vi "Target Startup Value Check.vi"(8 "error in (no error)":errorcluster) -> (0 "Ok to run?":bool)   [LabVIEW 2018]
panel:
  out "GRF Gain":bool
  out "Max Current":bool
  out "PCA weights":bool
  out "Logging Filename":bool
  out "Logging duration":bool
  out "Period Time":bool
  out "Bias":bool
  out "Current Rate":bool
  out "Mass":bool
  out "fc":bool
  out "HSD dF Thr":bool
  out "HSD F Thr":bool
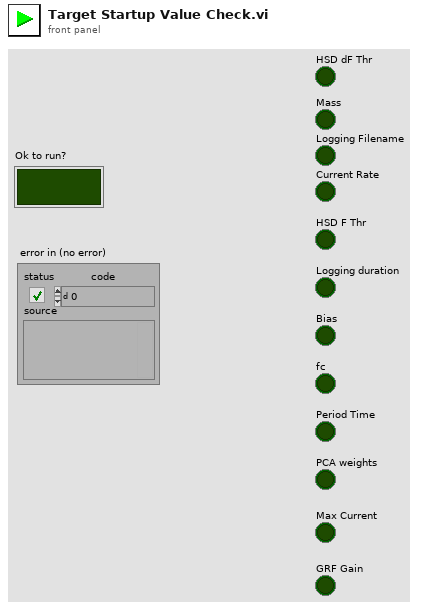
[diagram p1: front panel]
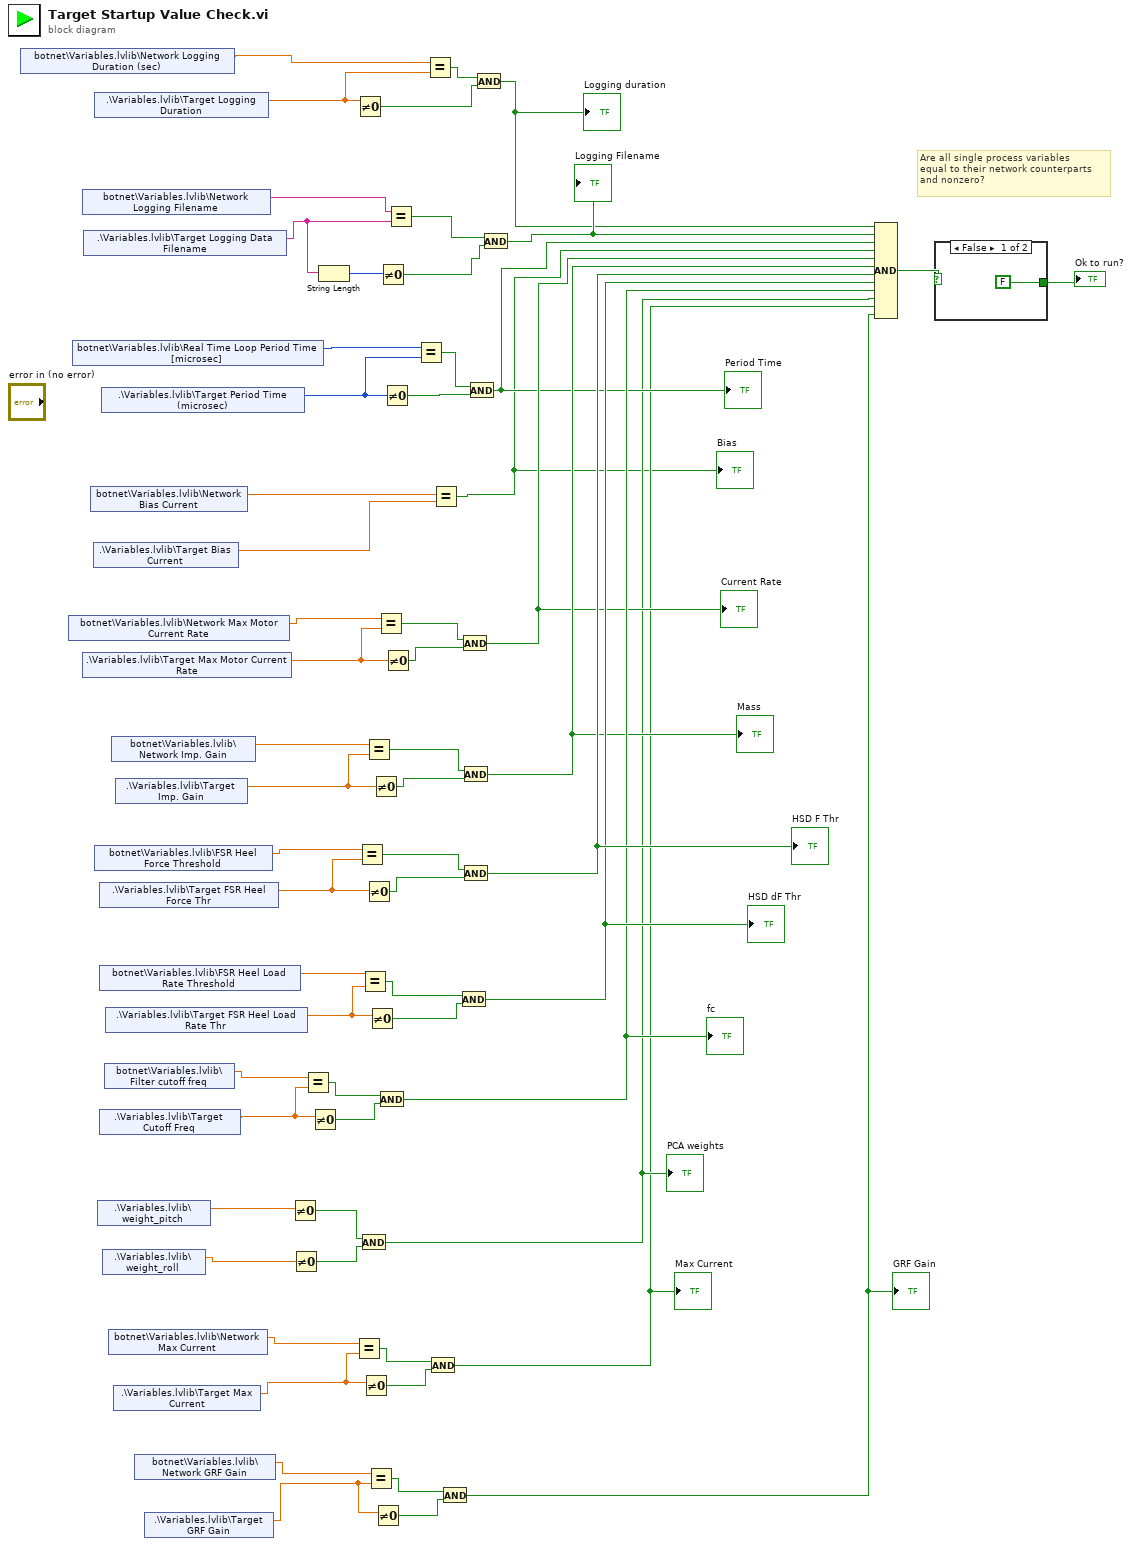
[diagram p0: block diagram]
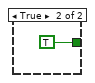
[diagram p2: hidden frame]
diagram:
  # "Are all single process variables \nequal to their network counterparts \nand nonzero?"
  n1 = shared-variable "botnet\\Variables.lvlib\\Network Logging Duration (sec)"() -> (w2:dbl)  [unwired: 1 in, 1 out]
  n2 = shared-variable "botnet\\Variables.lvlib\\Network Max Motor Current Rate"() -> (w50:dbl)  [unwired: 1 in, 1 out]
  n3 = shared-variable "botnet\\Variables.lvlib\\Real Time Loop Period Time [microsec]"() -> (w59:u32)  [unwired: 1 in, 1 out]
  n4 = shared-variable "botnet\\Variables.lvlib\\Network Logging Filename"() -> (w60:string)  [unwired: 1 in, 1 out]
  n5 = shared-variable ".\\Variables.lvlib\\Target Max Motor Current Rate"() -> (w51:dbl)  [unwired: 1 in, 1 out]
  n6 = shared-variable ".\\Variables.lvlib\\Target Logging Data Filename"() -> (w55:string)  [unwired: 1 in, 1 out]
  n7 = shared-variable "botnet\\Variables.lvlib\\Network Bias Current"() -> (w57:dbl)  [unwired: 1 in, 1 out]
  n8 = shared-variable ".\\Variables.lvlib\\Target Bias Current"() -> (w56:dbl)  [unwired: 1 in, 1 out]
  n9 = shared-variable ".\\Variables.lvlib\\Target Logging Duration"() -> (w61:dbl)  [unwired: 1 in, 1 out]
  n10 = shared-variable "botnet\\Variables.lvlib\\FSR Heel Force Threshold"() -> (w47:dbl)  [unwired: 1 in, 1 out]
  n11 = shared-variable ".\\Variables.lvlib\\weight_pitch"() -> (w37:dbl)  [unwired: 1 in, 1 out]
  n12 = shared-variable ".\\Variables.lvlib\\Target FSR Heel Force Thr"() -> (w46:dbl)  [unwired: 1 in, 1 out]
  n13 = shared-variable "botnet\\Variables.lvlib\\FSR Heel Load Rate Threshold"() -> (w45:dbl)  [unwired: 1 in, 1 out]
  n14 = shared-variable ".\\Variables.lvlib\\Target Cutoff Freq"() -> (w35:dbl)  [unwired: 1 in, 1 out]
  n15 = shared-variable ".\\Variables.lvlib\\Target Period Time (microsec)"() -> (w58:u16)  [unwired: 1 in, 1 out]
  n16 = shared-variable ".\\Variables.lvlib\\weight_roll"() -> (w36:dbl)  [unwired: 1 in, 1 out]
  n17 = shared-variable "botnet\\Variables.lvlib\\Filter cutoff freq"() -> (w34:dbl)  [unwired: 1 in, 1 out]
  n18 = shared-variable ".\\Variables.lvlib\\Target FSR Heel Load Rate Thr"() -> (w44:dbl)  [unwired: 1 in, 1 out]
  n19 = shared-variable "botnet\\Variables.lvlib\\Network Max Current"() -> (w10:dbl)  [unwired: 1 in, 1 out]
  n20 = shared-variable "botnet\\Variables.lvlib\\Network Imp. Gain"() -> (w49:dbl)  [unwired: 1 in, 1 out]
  n21 = shared-variable ".\\Variables.lvlib\\Target Max Current"() -> (w9:dbl)  [unwired: 1 in, 1 out]
  n22 = shared-variable ".\\Variables.lvlib\\Target Imp. Gain"() -> (w48:dbl)  [unwired: 1 in, 1 out]
  n23 = shared-variable "botnet\\Variables.lvlib\\Network GRF Gain"() -> (w5:dbl)  [unwired: 1 in, 1 out]
  n24 = shared-variable ".\\Variables.lvlib\\Target GRF Gain"() -> (w4:dbl)  [unwired: 1 in, 1 out]
  n25 = Not Equal To 0?(x=w37) -> (x != 0?=w15:bool)
  n26 = Not Equal To 0?(x=w36) -> (x != 0?=w14:bool)
  n27 = Equal?(x=w34, y=w35) -> (x = y?=w33:bool)
  n28 = Not Equal To 0?(x=w35) -> (x != 0?=w32:bool)
  n29 = String Length(string=w55) -> (length=w54:i32)
  n30 = Equal?(x=w10, y=w9) -> (x = y?=w12:bool)
  n31 = Not Equal To 0?(x=w61) -> (x != 0?=w18:bool)
  n32 = Equal?(x=w47, y=w46) -> (x = y?=w43:bool)
  n33 = And(x=w15, y=w14) -> (x .and. y?=w13:bool)
  "PCA weights" <- w13
  n34 = Equal?(x=w45, y=w44) -> (x = y?=w41:bool)
  n35 = Not Equal To 0?(x=w9) -> (x != 0?=w11:bool)
  n36 = Equal?(x=w49, y=w48) -> (x = y?=w30:bool)
  n37 = Not Equal To 0?(x=w46) -> (x != 0?=w42:bool)
  n38 = Equal?(x=w5, y=w4) -> (x = y?=w7:bool)
  n39 = Not Equal To 0?(x=w44) -> (x != 0?=w40:bool)
  n40 = Not Equal To 0?(x=w48) -> (x != 0?=w29:bool)
  n41 = Not Equal To 0?(x=w4) -> (x != 0?=w6:bool)
  n42 = Equal?(x=w50, y=w51) -> (x = y?=w27:bool)
  n43 = And(x=w33, y=w32) -> (x .and. y?=w31:bool)
  "fc" <- w31
  n44 = Not Equal To 0?(x=w54) -> (x != 0?=w21:bool)
  n45 = Not Equal To 0?(x=w58) -> (x != 0?=w23:bool)
  n46 = Not Equal To 0?(x=w51) -> (x != 0?=w26:bool)
  n47 = Equal?(x=w60, y=w55) -> (x = y?=w20:bool)
  n48 = Equal?(x=w59, y=w58) -> (x = y?=w24:bool)
  n49 = Equal?(x=w2, y=w61) -> (x = y?=w19:bool)
  n50 = And(x=w12, y=w11) -> (x .and. y?=w8:bool)
  "Max Current" <- w8
  n51 = Equal?(x=w57, y=w56) -> (x = y?=w1:bool)
  "Bias" <- w1
  n52 = And(x=w7, y=w6) -> (x .and. y?=w3:bool)
  "GRF Gain" <- w3
  n53 = And(x=w41, y=w40) -> (x .and. y?=w38:bool)
  "HSD dF Thr" <- w38
  n54 = And(x=w27, y=w26) -> (x .and. y?=w25:bool)
  "Current Rate" <- w25
  n55 = And(x=w30, y=w29) -> (x .and. y?=w28:bool)
  "Mass" <- w28
  n56 = And(x=w43, y=w42) -> (x .and. y?=w39:bool)
  "HSD F Thr" <- w39
  n57 = And(x=w24, y=w23) -> (x .and. y?=w16:bool)
  "Period Time" <- w16
  n58 = And(x=w19, y=w18) -> (x .and. y?=w17:bool)
  "Logging duration" <- w17
  n59 = And(x=w20, y=w21) -> (x .and. y?=w22:bool)
  "Logging Filename" <- w22
  n60 = Compound Arithmetic op=AND(w17, w22, w16, w1, w25, w28, w39, w38, w31, w13, w8, w3) -> (w53:bool)
  n61 = case shown="False" w53 {
    tunnel: [FALSE TRUE] -> w52
    frame False {
    }
    frame True {
    }
  }
  "Ok to run?" <- w52
